vi "Guardar Datos.vi"(9 "Intervalo de archivos (seg)":dbl=10.0, 10 "Data folder":path, 11 "Data":T1(array[cluster])) -> ()   [LabVIEW 2012]
uses:
  <vilib>/Utility/file.llb/Write To Spreadsheet File (string).vi
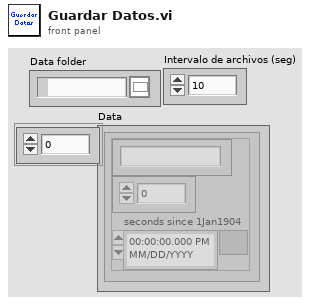
[diagram p1: front panel]
types:
  T1 = cluster{"String":string, "Numeric Control":dbl, "seconds since 1Jan1904":timestamp}[]
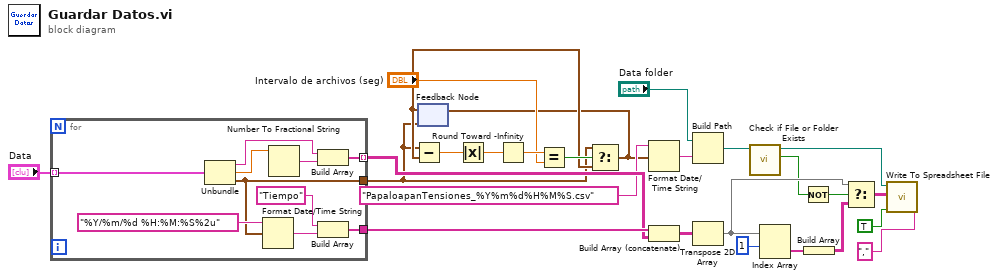
[diagram p0: block diagram]
diagram:
  n1 = for {
    tunnel: "Data" -> [w36] mode=indexing
    tunnel: [w32] -> w18 mode=indexing
    tunnel: [w28] -> w19
    tunnel: [w27] -> w2
    n2 = Unbundle(w36) -> ("String"=w33:string, "Numeric Control"=w34:dbl, "seconds since 1Jan1904"=w27:timestamp)
    n3 = Format Date/Time String(time format string (%c)="%Y/%m/%d %H:%M:%S%2u", seconds (now)=w27) -> (date/time string=w29:string)  [unwired: 1 in]
    n4 = Number To Fractional String(number=w34) -> (F-format string=w31:string)  [unwired: 3 in]
    n5 = Build Array(w33, w31) -> (w32:string[])
    n6 = Build Array("Tiempo" ("time format string (%c)"), w29) -> (w28:string[])
  }
  n7 = feedback #1(w2) -> (w21:timestamp)
  n8 = Subtract(x=w2, y=w21) -> (x-y=w22:dbl)
  n9 = Absolute Value(x=w22) -> (abs(x)=w25:dbl)
  n10 = Round Toward -Infinity(1:w25) -> (0:w26:dbl)
  n11 = Equal?(x=w26, y="Intervalo de archivos (seg)") -> (x = y?=w23:bool)
  n12 = Select(t=w2, s=w23, f=w21) -> (s? t:f=w1:timestamp)
  n13 = feedback-in #1(w1) -> ()
  n14 = Format Date/Time String(time format string (%c)="PapaloapanTensiones_%Y%m%d%H%M%S.csv", seconds (now)=w1) -> (date/time string=w14:string)  [unwired: 1 in]
  n15 = Build Array (concatenate)(w19, w18) -> (w20:string[][])
  n16 = Build Path(base path="Data folder", name or relative path=w14) -> (appended path=w6:path)
  n17 = Transpose 2D Array(2D array=w20) -> (transposed array=w10:string[][])
  n18 = call <vilib>:"Check if File or Folder Exists.vi"("path"=w6) -> ("file or folder exists?"=w5:bool, "dup path"=w3:path)  [unwired: 8 in, 1 out]
  n19 = Index Array(array=w10, index (row)=1) -> (element=w9:string[])  [unwired: 1 in]
  n20 = Not(x=w5) -> (.not. x?=w4:bool)
  n21 = Build Array(w9) -> (w8:string[][])
  n22 = Select(t=w10, s=w4, f=w8) -> (s? t:f=w7:string[][])
  n23 = call-poly <vilib>:"Write To Spreadsheet File.vi"("delimiter (\\t)"="," ("delimiter (\\t)"), "append to file? (new file:F)"=TRUE, "2D data"=w7, "file path (dialog if empty)"=w3) -> ()  [unwired: 4 in, 1 out]
